vi "Get Loop Synch Occurance.vi"(8 "Error In":errorcluster) -> (0 "Error Out":errorcluster, 3 "Loop Synch Occourance":refnum<k4>)   [LabVIEW 2014]
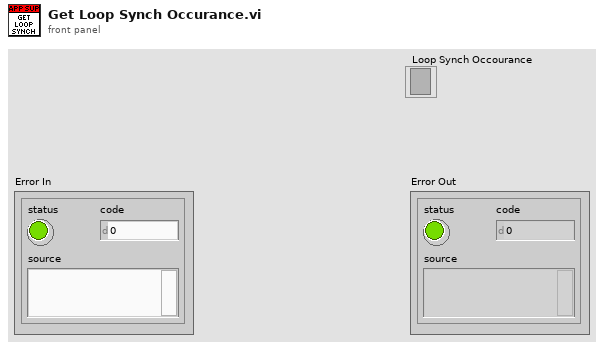
[diagram p1: front panel]
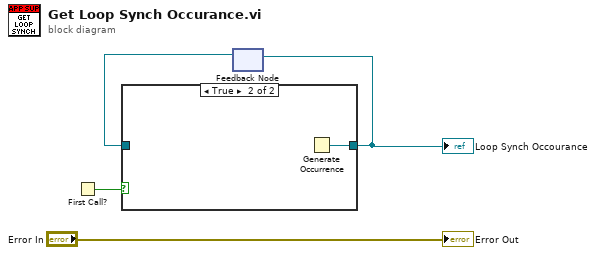
[diagram p0: block diagram]
diagram:
  n1 = First Call?() -> (First Call?: T/F=w3:bool)
  n2 = feedback #1() -> (w1:refnum<k4>)  [unwired: 1 in]
  n3 = case shown="True" w3 {
    tunnel: [w5 w6] -> w2
    tunnel: w1 -> [w5 _]
    frame False {
    }
    frame True {
      n4 = Generate Occurrence() -> (w6:refnum<k4>)
    }
  }
  "Loop Synch Occourance" <- w2
  n5 = feedback-in #1(w2) -> ()
  "Error Out" <- "Error In"
